vi "认识顺序结构.vi"() -> ()   [LabVIEW 2018]
panel:
  out "布尔 3":bool
  out "布尔 2":bool
  out "布尔":bool
  out "字符串":string="顺序结构：按照事先编程，按顺序执行\n层叠式，平铺式\n"
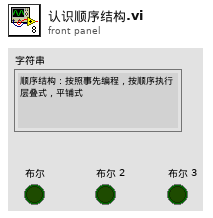
[diagram p1: front panel]
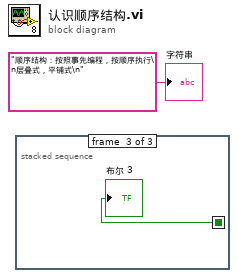
[diagram p0: block diagram]
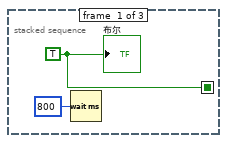
[diagram p2: hidden frame]
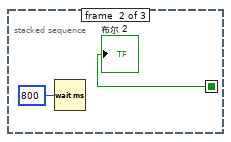
[diagram p3: hidden frame]
diagram:
  n1 = stacked-sequence {
    seq-local: [w3 _ _] -> [_ w5 w6]
    frame #0 {
      w3 = TRUE
      n2 = Wait (ms)(milliseconds to wait=u32 800 ("等待时间（毫秒）")) -> ()  [unwired: 1 out]
      "布尔" <- w3
    }
    frame #1 {
      n3 = Wait (ms)(milliseconds to wait=u32 800 ("等待时间（毫秒）")) -> ()  [unwired: 1 out]
      "布尔 2" <- w5
    }
    frame #2 {
      "布尔 3" <- w6
    }
  }
  "字符串" <- "顺序结构：按照事先编程，按顺序执行\n层叠式，平铺式\n"
